vi "grab and threshold.vi"() -> ()   [LabVIEW 2011]
uses:
  <userlib>/labvvis/New Image/New Image (RGBA).vi
  <userlib>/labvvis/labvvis.lvlib
panel:
  out "Error":string
  in  "stop":bool
  in  "Threshold":u8(slide)=128 scale=0.0..255.0
  out "Output":picture
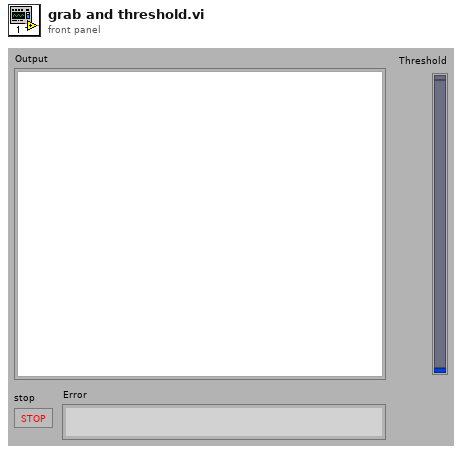
[diagram p1: front panel]
types:
  T1 = typedef "labvvis.lvlib/VVIS Image.ctl" = cluster{"Image ID":i16, "Channel ID":i16}
  T2 = typedef "imagedata.ctl" = cluster{"image type":i32, "image depth":i32, "image":u8[], "mask":u8[], "colors":u32[], "Rectangle":cluster{"left":i16, "top":i16, "right":i16, "bottom":i16}}
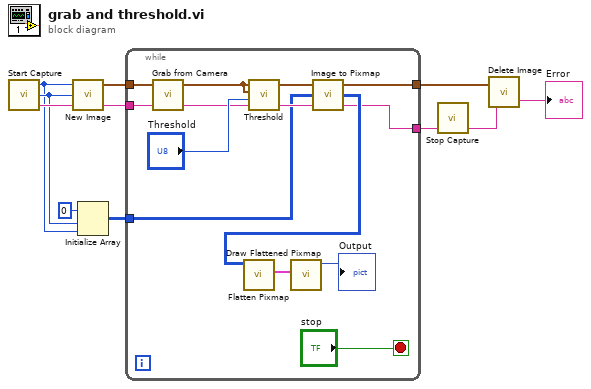
[diagram p0: block diagram]
diagram:
  n1 = call <userlib>:"Start Capture.vi"() -> ("Error"=w8:string, "Height"=w7:i32, "Width"=w6:i32)  [unwired: 3 in]
  n2 = call-poly <userlib>:"New Image.vi"("Error"=w8, "Height"=w7, "Width"=w6) -> ("Error"=w5:string, "VVIS Image"=w9:T1)  [unwired: 1 in]
  n3 = Initialize Array(0, w7, w6) -> (w10:i32[][])
  n4 = while {
    tunnel: w10 -> [w14]
    tunnel: w9 -> [w21]
    tunnel: w5 -> [w20]
    tunnel: [w15] -> w4
    tunnel: [w12] -> w3
    stop <- "stop" stop-if-true
    n5 = call <userlib>:"Grab from Camera.vi"("Error"=w20, "Image"=w21) -> ("Error"=w17:string, "Image"=w19:T1)  [unwired: 1 in, 1 out]
    n6 = call <userlib>:"Threshold.vi"("Error"=w17, "Threshold"="Threshold", "Output Image"=w19, "Input Image"=w19) -> ("Error"=w16:string, "Input Image"=w18:T1)  [unwired: 1 out]
    n7 = call <userlib>:"Image to Pixmap.vi"("Error"=w16, "Output Pixmap"=w14, "Image"=w18) -> ("Error"=w12:string, "Output Pixmap"=w13:u32[][], "Image"=w15:T1)
    n8 = call <vilib>:"Flatten Pixmap.vi"("24-bit pixmap"=w13) -> ("image data"=w25:T2)  [unwired: 10 in]
    n9 = call <vilib>:"Draw Flattened Pixmap.vi"("image data"=w25) -> ("new picture"=→"Output":picture)  [unwired: 8 in]
  }
  n10 = call <userlib>:"Stop Capture.vi"("Error"=w3) -> ("Error"=w2:string)  [unwired: 4 in]
  n11 = call <userlib>:"Delete Image.vi"("Error"=w2, "Image"=w4) -> ("Error"=→"Error":string)  [unwired: 1 in]
